vi "Agilent SNA Read Number of Points.vi"(6 "Channel":i8=1 min=1 max=99 step=1, 7 "Agilent SNA & SWP":T1, 8 "error in (no error)":errorcluster, 11 "VISA Resource Names":T2) -> (0 "error out":errorcluster, 2 "Number Points":i32, 3 "dup VISA Resource Names":T2)   [LabVIEW 2011]
doc: "This VI for the HP 8753B is used to read the number of stimulus points."
uses:
  TypeDefs/Agilent SNA VISA.ctl
  TypeDefs/Agilent SNA Instrument Info.ctl
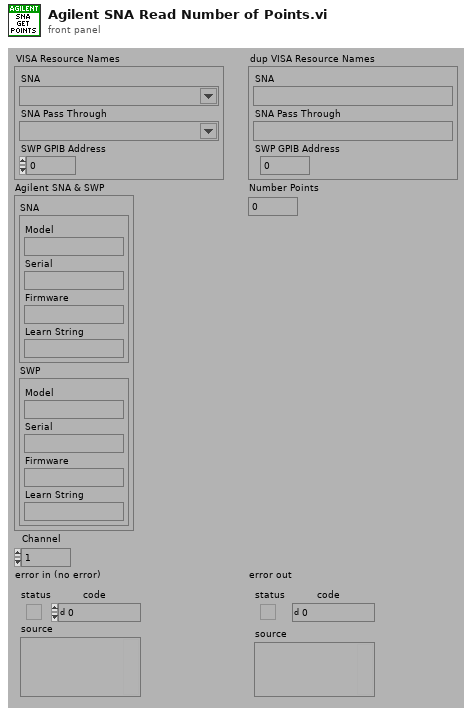
[diagram p1: front panel]
types:
  T1 = typedef "Agilent SNA Instrument Info.ctl" = cluster{"SNA":cluster{"Model":string, "Serial":string, "Firmware":string, "Learn String":string}, "SWP":cluster{"Model":string, "Serial":string, "Firmware":string, "Learn String":string}}
  T2 = typedef "Agilent SNA VISA.ctl" = cluster{"SNA":refnum<visa-resource-name>, "SNA Pass Through":refnum<visa-resource-name>, "SWP GPIB Address":i32}
  T3 = typedef "Agilent SNA Model.ctl" = enum16{"Not Supported", "8757X"}
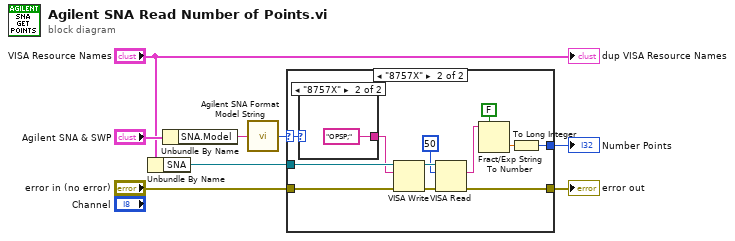
[diagram p0: block diagram]
diagram:
  n1 = Unbundle By Name("VISA Resource Names") -> ("SNA"=w1:refnum<visa-resource-name>)
  n2 = Unbundle By Name("Agilent SNA & SWP") -> ("SNA.Model"=w4:string)
  n3 = call "Agilent SNA Format Model String.vi"("Model String"=w4) -> ("Model"=w3:T3)
  n4 = case shown="\"8757X\"" w3 {
    selector: w3 -> [_ w10]
    tunnel: [w9 w21] -> w8
    tunnel: w1 -> [_ w20]
    tunnel: "error in (no error)" -> [w9 w19]
    tunnel: [_ w18] -> w6
    frame "Not Supported" {
    }
    frame "8757X" {
      n5 = case shown="\"8757X\"" w10 {
        tunnel: [_ "OPSP;"] -> w11
        frame "Not Supported" {
        }
        frame "8757X" {
        }
      }
      n6 = VISA Write(VISA resource name=w20, write buffer=w11, error in (no error)=w19) -> (VISA resource name out=w14:refnum<visa-resource-name>, error out=w17:errorcluster)  [unwired: 1 out]
      n7 = VISA Read(VISA resource name=w14, byte count=u32 50, error in (no error)=w17) -> (read buffer=w16:string, error out=w21:errorcluster)  [unwired: 2 out]
      n8 = Fract/Exp String To Number(use system decimal point (T)=FALSE, string=w16) -> (number=w15:dbl)  [unwired: 3 out]
      n9 = To Long Integer(number=w15) -> (32bit integer=w18:i32)
    }
  }
  "Number Points" <- w6
  "error out" <- w8
  "dup VISA Resource Names" <- "VISA Resource Names"
